vi "DeadReckoning (SubVI).vi"(6 "Theta_0":dbl, 7 "Robot Width":dbl, 8 "y0":dbl, 9 "x0":dbl, 10 "sL":i32, 11 "sR":i32) -> (0 "Theta Actual (rad)":dbl, 1 "Theta (rad)":dbl, 2 "y":dbl, 3 "x":dbl, 5 "sBar":dbl)   [LabVIEW 2017]
panel:
  out "Theta Waveform":dbl(graph)
  out "Waveform Chart":dbl(graph)
  # "VI Name: DeadReckoning (SubVI).vi\nAuthor: Steven Lee\n\nOnce provided with the required input values, this SubVI computes robot's x-y position and heading Theta."
  # "Use this theta for main loop shift register."
  # "Reference:\nUsing \"A Simpler Formula for Dead Reckoning\" in eqn [6]\nhttp://rossum.sourceforge.net/papers/DiffSteer/"
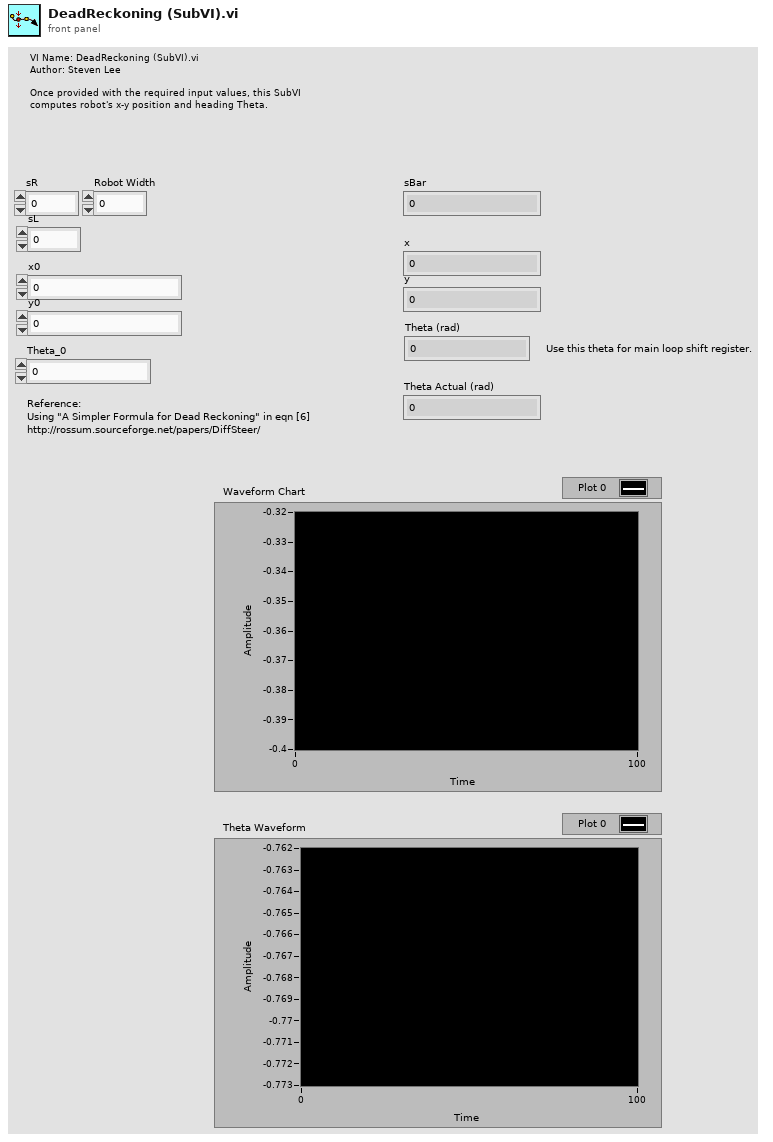
[diagram p1: front panel]
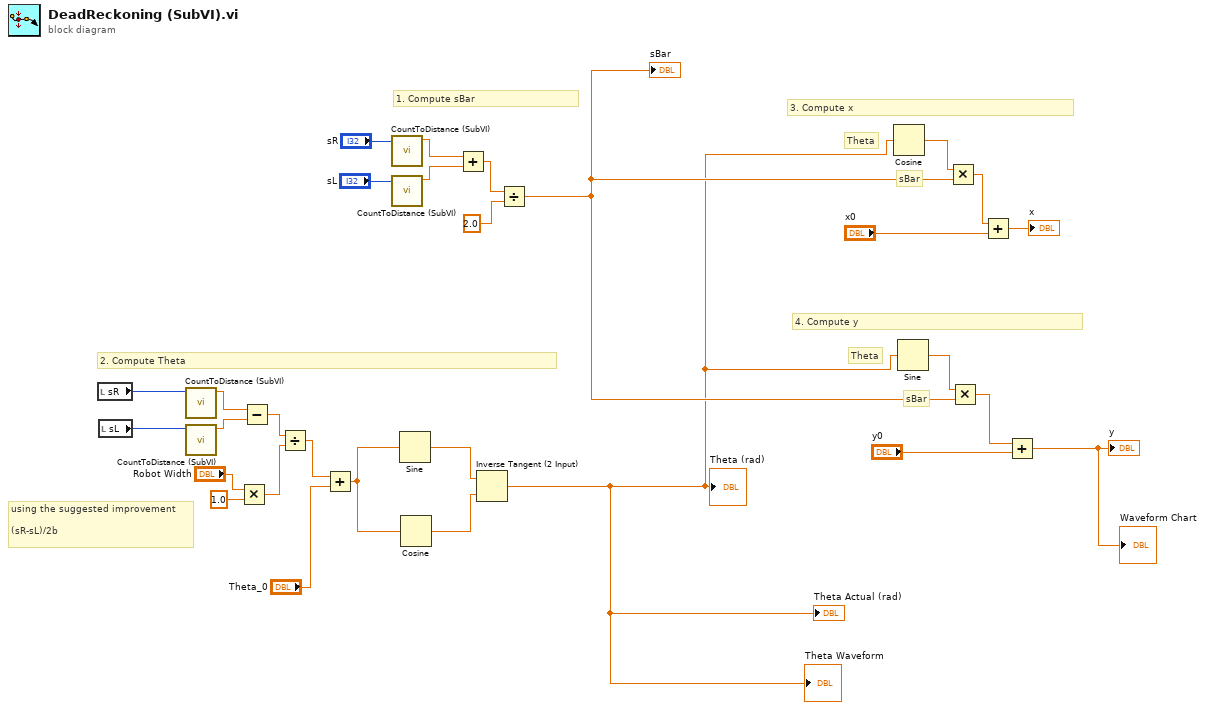
[diagram p0: block diagram]
diagram:
  # "using the suggested improvement\n\n(sR-sL)/2b"
  # "sBar"
  # "Theta"
  # "sBar"
  # "Theta"
  # "4. Compute y"
  # "3. Compute x"
  # "2. Compute Theta"
  # "1. Compute sBar"
  n1 = local read "sR"() -> (w12:i32)
  n2 = local read "sL"() -> (w10:i32)
  n3 = call "CountToDistance (SubVI).vi"("Counter Value"=w12) -> ("Total Distance Travelled (m)"=w11:dbl)  [unwired: 10 in]
  n4 = call "CountToDistance (SubVI).vi"("Counter Value"=w10) -> ("Total Distance Travelled (m)"=w9:dbl)  [unwired: 10 in]
  n5 = Multiply(x="Robot Width", y=1.0) -> (x*y=w1:dbl)
  n6 = Subtract(x=w11, y=w9) -> (x-y=w27:dbl)
  n7 = Divide(x=w27, y=w1) -> (x/y=w26:dbl)
  n8 = Add(x=w26, y="Theta_0") -> (x+y=w8:dbl)
  n9 = call "CountToDistance (SubVI).vi"("Counter Value"="sR") -> ("Total Distance Travelled (m)"=w15:dbl)  [unwired: 10 in]
  n10 = call "CountToDistance (SubVI).vi"("Counter Value"="sL") -> ("Total Distance Travelled (m)"=w13:dbl)  [unwired: 10 in]
  n11 = Sine(x=w8) -> (sin(x)=w7:dbl)
  n12 = Cosine(x=w8) -> (cos(x)=w6:dbl)
  n13 = Add(x=w15, y=w13) -> (x+y=w29:dbl)
  n14 = Inverse Tangent (2 Input)(1:w6, 2:w7) -> (0:w5:dbl)
  "Theta Actual (rad)" <- w5
  "Theta Waveform" <- w5
  "Theta (rad)" <- w5
  n15 = Divide(x=w29, y=2.0) -> (x/y=w17:dbl)
  "sBar" <- w17
  n16 = Cosine(x=w5) -> (cos(x)=w21:dbl)
  n17 = Sine(x=w5) -> (sin(x)=w20:dbl)
  n18 = Multiply(x=w21, y=w17) -> (x*y=w19:dbl)
  n19 = Multiply(x=w20, y=w17) -> (x*y=w18:dbl)
  n20 = Add(x=w19, y="x0") -> (x+y=→"x":dbl)
  n21 = Add(x=w18, y="y0") -> (x+y=→"y" →"Waveform Chart":dbl)
